vi "SL TAGS Add-Update Single Tag Property.vi"(8 "error in (no error)":errorcluster, 10 "Tag Property In":T1 caption="Property", 11 "Tag Ref In":T2={"Class Properties"={"Class Data Type"=enum."Double", "Name"="", "Description"="", "Interpolation Method"=enum."linear", "Unit of Measure"=enum."Hour", "Maximum Interpolation"="", "Role"=enum."Supervisor"}, "SL Tag"=refnum, "SystemLink Cluster"={"Path"="", "Data Type"=enum."Double", "Value"=variant, "Time Stamp"=timestamp(0 s since 1904-01-01)}, "Class Value"=variant}) -> (0 "error out":errorcluster, 2 "Tag Property Out":T1 caption="Property", 3 "Tag Ref Out":T2={"Class Properties"={"Class Data Type"=enum."Double", "Name"="", "Description"="", "Interpolation Method"=enum."linear", "Unit of Measure"=enum."Hour", "Maximum Interpolation"="", "Role"=enum."Supervisor"}, "SL Tag"=refnum, "SystemLink Cluster"={"Path"="", "Data Type"=enum."Double", "Value"=variant, "Time Stamp"=timestamp(0 s since 1904-01-01)}, "Class Value"=variant})   [LabVIEW 2017, in "EEISysLink.lvclass"]
doc: "Will check the tag properties for \"key\". If found it will update and if not it will add the property. Note: This updates the single tag copy of properties. \n\nJames Tillett P.E.\nEndeavor Engineering Inc.\nwww.endeavoreng.com"
uses:
  EEISysLink.lvclass
  <vilib>/Skyline/Tag/Shared/typedefs/TagProperty.ctl
  Controls/SL Tag.ctl
  <vilib>/Skyline/Tag/Wrapper/Wrapper_class/NI Skyline Tag.lvclass
  Controls/SL Tag Properties.ctl
  Controls/SL Tag Data Type.ctl
  Controls/SL Tag Interpolation Method.ctl
  Controls/SL Tag Unit of Measure.ctl
  Controls/SL Tag Type.ctl
  <vilib>/Skyline/Tag/Shared/typedefs/Tag Cluster.ctl
  <vilib>/Skyline/Tag/Shared/typedefs/DataType.ctl
  <vilib>/Skyline/Tag/Shared/NI Skyline Tag.lvlib
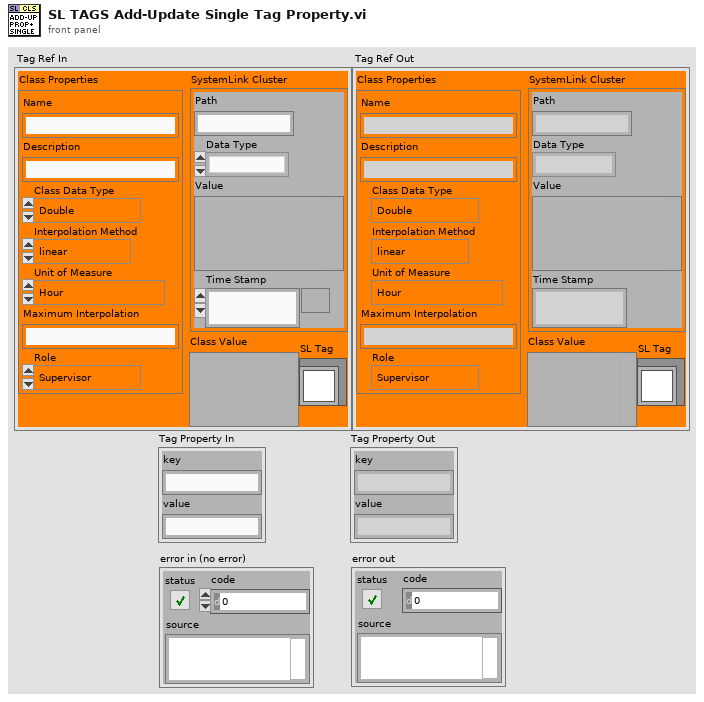
[diagram p1: front panel]
types:
  T1 = typedef "NI Skyline Tag.lvlib/TagProperty.ctl" = cluster{"key":string, "value":string}
  T2 = typedef "EEISysLink.lvclass/SL Tag.ctl" = cluster{"Class Properties":T3, "SL Tag":refnum<class "NI Skyline Tag.lvclass">, "SystemLink Cluster":T8, "Class Value":variant}
  T3 = typedef "EEISysLink.lvclass/SL Tag Properties.ctl" = cluster{"Class Data Type":T4, "Name":string, "Description":string, "Interpolation Method":T5, "Unit of Measure":T6, "Maximum Interpolation":string, "Role":T7}
  T4 = typedef "EEISysLink.lvclass/SL Tag Data Type.ctl" = enum16{"Double", "Integer", "String", "Boolean", "Waveform"}
  T5 = typedef "EEISysLink.lvclass/SL Tag Interpolation Method.ctl" = enum16{"linear", "pilinear", "step"}
  T6 = typedef "EEISysLink.lvclass/SL Tag Unit of Measure.ctl" = enum16{"no units", "Second", "Hour", "Minute", "Day", "Year", "Month", "Week", "Foot", "Yard", "Meter", "Centimeter", "Inch", "Mile", "Nautical Mile", "Miles per Hour", "Meters per second", "Square meter", "Cubic meter", "Cubic centimeter", "Cubic inch", "Liter", "Gallon", "Gallons dry US", "Gallon UK", "Percent", "Revolutions per minute", "Revolution", "Degree angle", "Astronomical Unit", "Atom", "Atomic mass", "Bar", "Byte", "C (speed of light)", "Curie", "Decibel", "Electron Volt", "Ounce", "Knot", "G", "Grade", "Are", "Hectare", "Faraday", "Franklin", "Gilbert", "Erg", "Lambert", "Maxwell", "Gauss", "Electron mass", "Kilogram force", "Pound force", "Rad", "Centiradian", "Sphere", "Mach", "Fluid Ounces", "Fluid Ounces UK", "Fahrenheit", "Celsius", "Kelvin", "Rankine", "Gram", "Kilogram", "Pound", "Short/US Ton", "Long/UK ton", "Metric ton", "Mole", "Pounds per square inch", "Inches water column", "Torr", "Millitorr", "Millimeter mercury", "Inches mercury", "Bar (2)", "Atmosphere", "Pascal", "Watt", "kiloWatt", "Horsepower", "Kilowatt Hour", "British thermal units", "Millions of BTU", "Ampere", "Candela", "Radian", "Steradian", "Bit", "Hertz", "Newton", "Joule", "Coulomb", "Volt", "Farad", "Ohm", "Siemens", "Weber", "Tesla", "Henry", "Lumen", "Lux", "Becqueral", "Gray", "Sievert", "Katal", "Angstrom", "Light Year", "Parsec", "Point", "Pixel", "Dyne", "Kilogram force (2)", "Pound force (2)", "Rem", "Rutherford", "Roentgen"}
  T7 = typedef "EEISysLink.lvclass/SL Tag Type.ctl" = enum16{"All", "Supervisor", "Worker"}
  T8 = typedef "NI Skyline Tag.lvlib/Tag Cluster.ctl" = cluster{"Path":string, "Data Type":T9, "Value":variant, "Time Stamp":timestamp}
  T9 = typedef "NI Skyline Tag.lvlib/DataType.ctl" = enum32{"Double", "Integer", "String"}
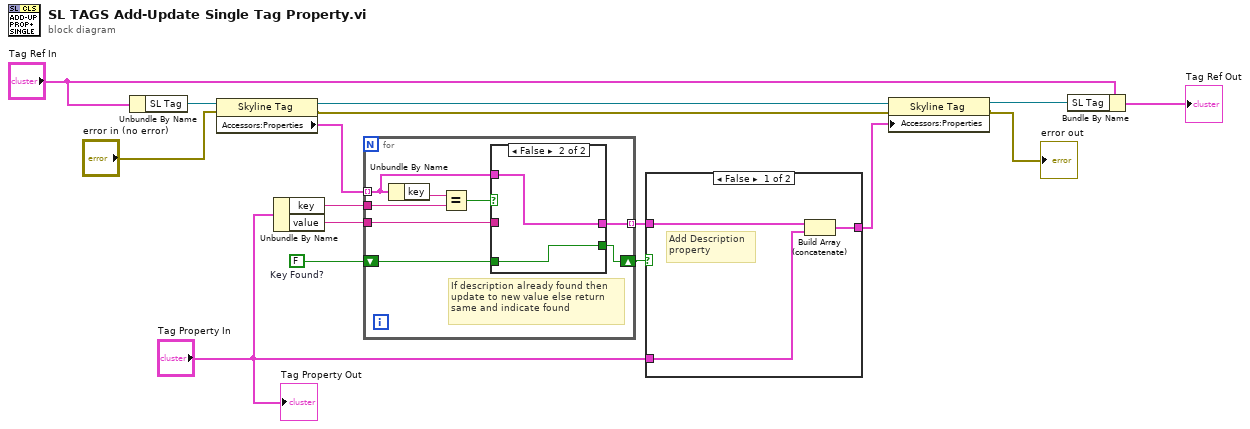
[diagram p0: block diagram]
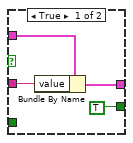
[diagram p3: hidden frame]
diagram:
  w14 = FALSE  # Key Found?
  n1 = Unbundle By Name("Tag Ref In") -> ("SL Tag"=w8:refnum<class "NI Skyline Tag.lvclass">)
  n2 = property on="Property Node" class="Skyline Tag"(reference=w8, error in="error in (no error)") -> (reference out=w5:refnum<class "NI Skyline Tag.lvclass">, error out=w4:errorcluster, "Accessors:Properties"=w6:T1[])
  n3 = Unbundle By Name("Tag Property In") -> ("key"=w13:string, "value"=w12:string)
  n4 = for {
    tunnel: w6 -> [w24] mode=indexing
    shift-right: [w22] -> w15
    shift-left: w14 -> [w23]
    tunnel: [w21] -> w16 mode=indexing
    tunnel: w13 -> [w19]
    tunnel: w12 -> [w18]
    # "If description already found then\nupdate to new value else return\nsame and indicate found"
    n5 = Unbundle By Name(w24) -> ("key"=w20:string)
    n6 = Equal?(x=w20, y=w19) -> (x = y?=w17:bool)
    n7 = case shown="False" w17 {
      tunnel: w24 -> [w28 w30]
      tunnel: w18 -> [w27 _]
      tunnel: [w26 w30] -> w21
      tunnel: w23 -> [_ w29]
      tunnel: [TRUE w29] -> w22
      frame True {
        n8 = Bundle By Name(cluster=w28, "value"=w27) -> (w26:T1)
      }
      frame False {
      }
    }
  }
  n9 = case shown="False" w15 {
    tunnel: w16 -> [w33 w34]
    tunnel: [w32 w34] -> w1
    tunnel: "Tag Property In" -> [w31 _]
    frame False {
      # "Add Description\nproperty"
      n10 = Build Array (concatenate)(w33, w31) -> (w32:T1[])
    }
    frame True {
      # "Description property already\nexists"
    }
  }
  n11 = property on="Property Node" class="Skyline Tag"(reference=w5, error in=w4, "Accessors:Properties"=w1) -> (reference out=w3:refnum<class "NI Skyline Tag.lvclass">, error out=→"error out":errorcluster)
  n12 = Bundle By Name(cluster="Tag Ref In", "SL Tag"=w3) -> (→"Tag Ref Out":T2)
  "Tag Property Out" <- "Tag Property In"
